vi "Graphics-Annotate With Image.vi"(0 "XYGraph in":refnum<vi>, 1 "Font size":i16=24, 5 "picture in":picture, 7 "Val":string, 9 "X":dbl, 11 "Y":dbl) -> (4 "XYGraph out":refnum<vi>, 6 "picture out":picture)   [LabVIEW 2020]
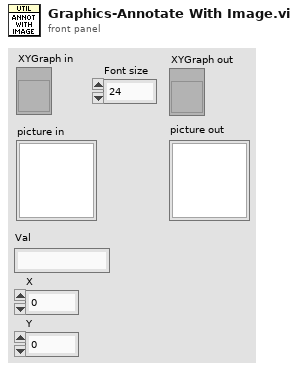
[diagram p1: front panel]
types:
  T1 = cluster{"Font Name:":string, "Size":i16, "Strikeout?":bool, "Italic?":bool, "Underline?":bool, "Outline?":bool, "Shadow?":bool, "Bold?":bool}
  T2 = enum16{"User-specified Font", "Application Font", "System Font", "Dialog Font"}
  T3 = cluster{"horizontal":enum16{"left", "center", "right"}, "vertical":enum16{"top", "center", "bottom"}}
  T4 = typedef "LVPoint32TypeDef.ctl" = cluster{"Horizontal":i32, "Vertical":i32}
  T5 = typedef "LVRectTypeDef.ctl" = cluster{"Left":i16, "Top":i16, "Right":i16, "Bottom":i16}
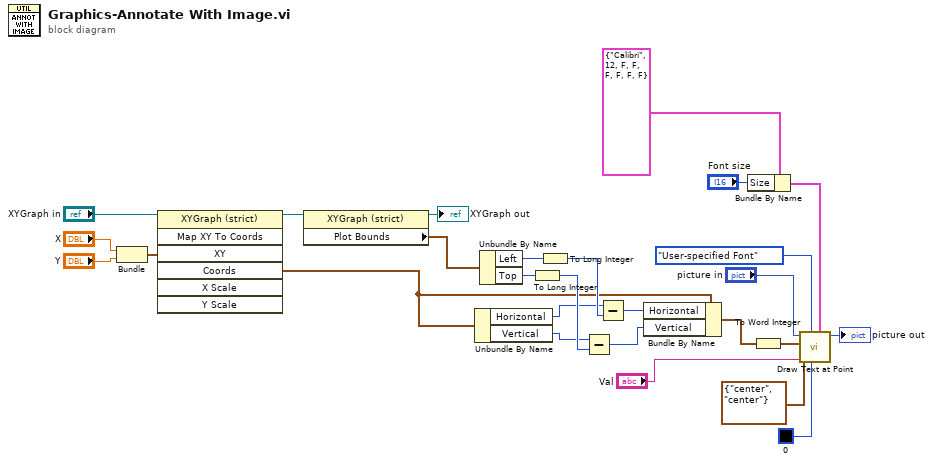
[diagram p0: block diagram]
diagram:
  n1 = Bundle("X"="X", "Y"="Y") -> (w27:cluster{"X":dbl, "Y":dbl})  [unwired: 1 in]
  n2 = invoke on="Invoke Node" class="XYGraph (strict)" method="Map XY To Coords"(reference="XYGraph in", "XY"=w27) -> (reference out=w5:refnum<vi>, "Coords"=w3:T4)  [unwired: 5 in, 5 out]
  n3 = property on="Property Node" class="XYGraph (strict)"(reference=w5) -> (reference out=→"XYGraph out":refnum<vi>, "Plot Bounds"=w23:T5)  [unwired: 1 in, 1 out]
  n4 = Unbundle By Name(w3) -> ("Horizontal"=w17:i32, "Vertical"=w18:i32)
  n5 = Unbundle By Name(w23) -> ("Left"=w15:i16, "Top"=w16:i16)
  n6 = To Long Integer(number=w16) -> (32bit integer=w22:i32)
  n7 = To Long Integer(number=w15) -> (32bit integer=w21:i32)
  n8 = Subtract(x=w18, y=w22) -> (x-y=w20:i32)
  n9 = Subtract(x=w17, y=w21) -> (x-y=w19:i32)
  n10 = Bundle By Name(cluster=w3, "Horizontal"=w19, "Vertical"=w20) -> (w7:T4)
  n11 = Bundle By Name(cluster=T1 {"Font Name:"="Calibri", "Size"=12, "Strikeout?"=FALSE, "Italic?"=FALSE, "Underline?"=FALSE, "Outline?"=FALSE, "Shadow?"=FALSE, "Bold?"=FALSE} ("[user-specified font]"), "Size"="Font size") -> (w9:T1)
  n12 = To Word Integer(number=w7) -> (16bit integer=w6:cluster{"Horizontal":i16, "Vertical":i16})
  n13 = call <vilib>:"Draw Text at Point.vi"("[user-specified font]"=w9, "text color(black)"=u32 0, "desired font(Application)"=T2."User-specified Font", "text"="Val", "alignment(left, top)"=T3 {"horizontal"=enum."center", "vertical"=enum."center"}, "origin"=w6, "picture"="picture in") -> ("new picture"=→"picture out":picture)  [unwired: 3 in, 1 out]
